vi "ME35.vi"() -> ()   [LabVIEW 2020]
panel:
  in  "Tab Control":T1(tab)
  in  "ports":bool
  in  "Prefs":bool
  in  "FileUpload":bool
  in  "VI Examples":u16(ring) items=["01 Controls and Indicators.vi", "02 Tools, Colors, and Clicks.vi", "03 Charts.vi", "04 Loops.vi", "05 Graphs.vi", "06 Shift Registers.vi", "07 Arrays.vi", "08 Strings.vi", "09 Clusters.vi", "10 Rings, Strings, and Tables.vi", "11 Execution Order.vi", "12 Events.vi", "13 Case Structures.vi", "14 Saving and Reading Files.vi", "15 Messing with Time.vi", "16 JSON Packets.vi", "21 Talking Serial.vi", "22 RESTful API.vi", "23 Python Node.vi", "24 OS Commands.vi", "51 Simple Queues.vi", "52 Properties.vi", "53 Invoke.vi", "54 Occurences and more.vi", "55 Channels.vi", "56 Panels in panels.vi", "57 Scripting.vi", "71 MP_Reading a voltage.vi", "72 MP_Setting a servo.vi", "81 Arduino_Reading a voltage.vi", "82 Arduino_Setting a servo.vi", "91 WIO_Reading a voltage.vi", "92 WIO_Setting a Servo.vi"]
  in  "VIs":bool
  in  "rPi":bool
  in  "IP Address":string
  in  "WIO":bool
  in  "WIO Port":string(combo)
  in  "Connect":bool
  in  "Port":string(combo)
  out "Python version":string="3.9"
  out "OUTPUT CONSOLE":string
  in  "Home 2":bool
  in  "Prefs":T2={"Python version"="3.9", "arduino15"=path "", "arduino Lib"=path ""}
  in  "Home":bool
  # "ME35\nversion 0.1b02"
  # "This program uses python codes under the hood to talk over the serial port, over SSH, and to cameras.  You should using version 3.6 or later and should have pyserial installed."
  # "This is the path to your Arduino app.  Click on the folder icon and select the app."
  # "This is the path to your Arduinolibarry folder (typically in your documents folder)"
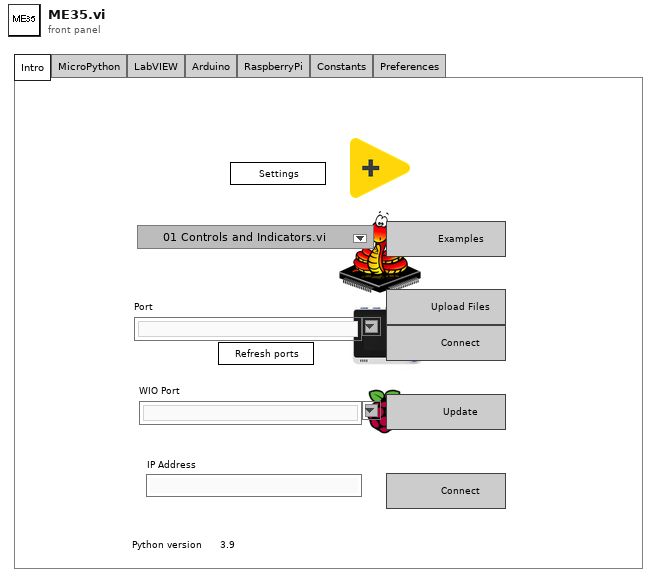
[diagram p1: front panel]
types:
  T1 = enum32{"Intro", "MicroPython", "LabVIEW", "Arduino", "RaspberryPi", "Constants", "Preferences"}
  T2 = cluster{"Python version":string, "arduino15":path, "arduino Lib":path}
  T3 = enum32{"Invalid", "Standard", "Closed", "Hidden", "Minimized", "Maximized"}
  T4 = typedef "Preferences.ctl" = cluster{"python":string, "arduino15":path, "arduino Lib":path}
  T5 = typedef "PythonCtrl.ctl" = cluster{"session":refnum<k35>, "PyPath":path}
  T6 = typedef "Arduino.ctl" = cluster{"Java":path, "Packages":path, "folder":path, "serial":string, "Console":string}
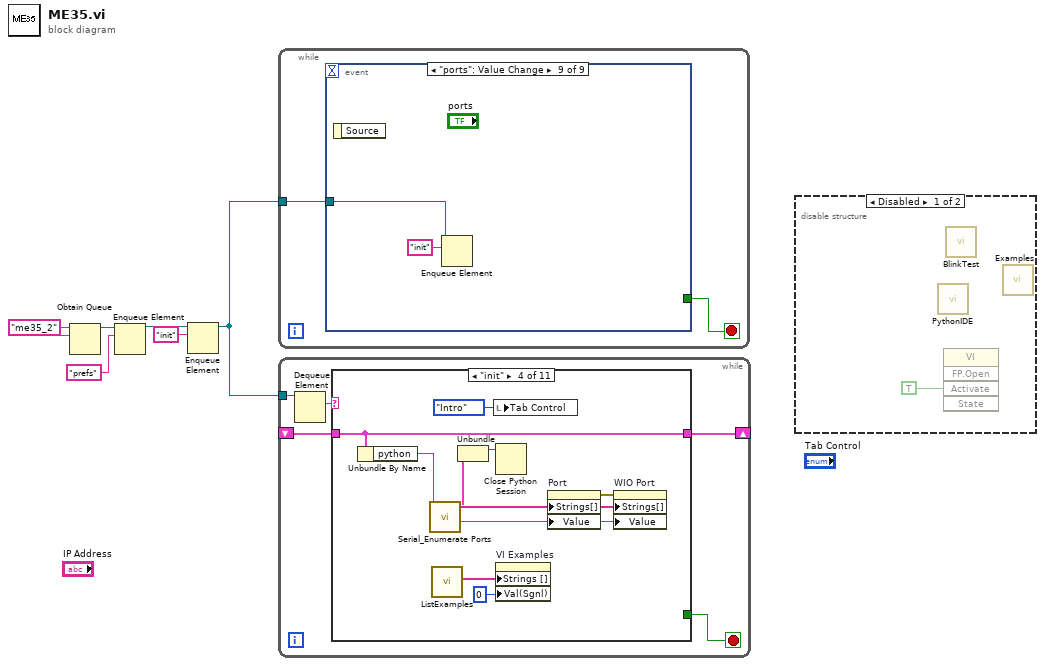
[diagram p0: block diagram]
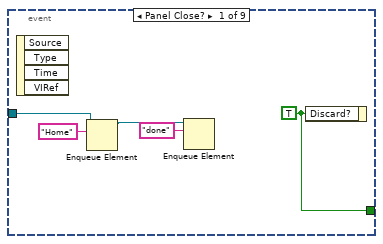
[diagram p3: hidden frame]
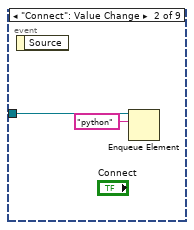
[diagram p4: hidden frame]
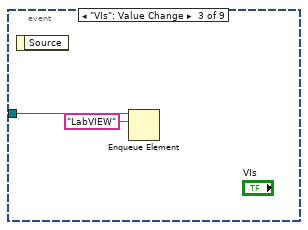
[diagram p5: hidden frame]
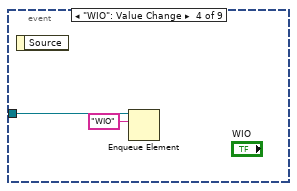
[diagram p6: hidden frame]
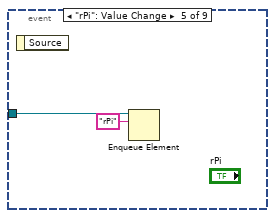
[diagram p7: hidden frame]
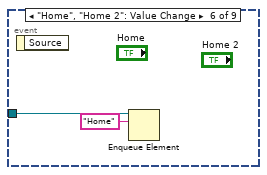
[diagram p8: hidden frame]
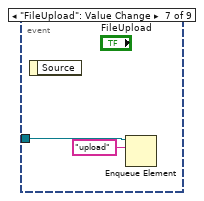
[diagram p9: hidden frame]
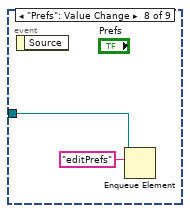
[diagram p10: hidden frame]
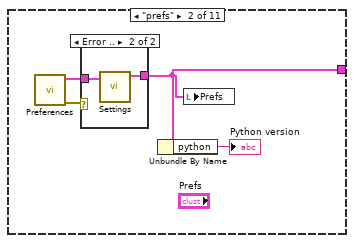
[diagram p12: hidden frame]
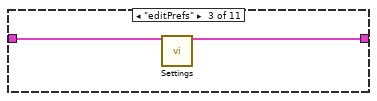
[diagram p14: hidden frame]
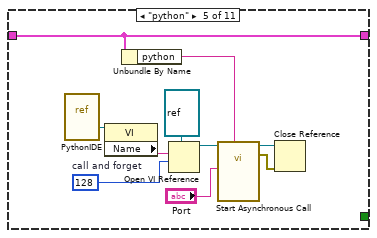
[diagram p15: hidden frame]
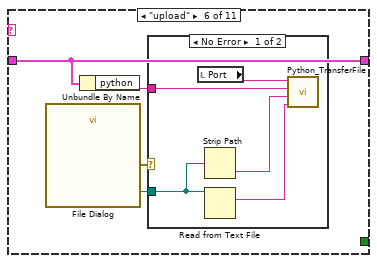
[diagram p16: hidden frame]
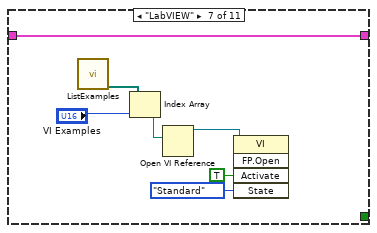
[diagram p18: hidden frame]
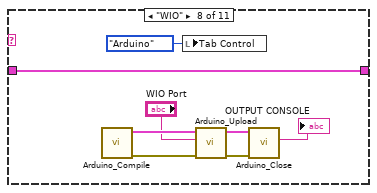
[diagram p19: hidden frame]
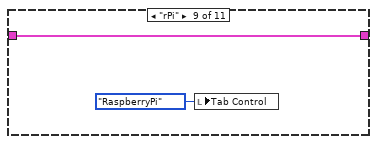
[diagram p20: hidden frame]
diagram:
  w6 = "me35_2" ("name (unnamed)")
  n1 = Obtain Queue(name (unnamed)=w6, element data type=w6) -> (queue out=w2:refnum<queue>)  [unwired: 3 in, 2 out]
  n2 = Enqueue Element(queue=w2, element="prefs") -> (queue out=w1:refnum<queue>)  [unwired: 2 in, 2 out]
  n3 = Enqueue Element(queue=w1, element="init") -> (queue out=w5:refnum<queue>)  [unwired: 2 in, 2 out]
  n4 = while {
    tunnel: w5 -> [w8]
    stop <- w7 stop-if-true
    n5 = event shown="[8] \"ports\": Value Change" {
      selector: _ -> [_ _ _ _ _ _ _ _ _]
      dyn-events: _ -> [_ _ _ _ _ _ _ _ _]
      timeout: _ -> [_ _ _ _ _ _ _ _ _]
      tunnel: w8 -> [w10 w15 w17 w19 w21 w23 w24 w26 w28]
      tunnel: [w13 _ _ _ _ _ _ _ _] -> w7
      event Panel Close? {
        w13 = TRUE ("Discard?")
        n6 = event-data() -> ()  [unwired: 1 in, 4 out]
        n7 = Enqueue Element(queue=w10, element="Home") -> (queue out=w9:refnum<queue>)  [unwired: 2 in, 2 out]
        n8 = Enqueue Element(queue=w9, element="done") -> ()  [unwired: 2 in, 3 out]
        n9 = event-data("Discard?"=w13) -> ()  [unwired: 1 in, 1 out]
      }
      event "Connect": Value Change {
        n10 = event-data() -> ()  [unwired: 1 in, 1 out]
        n11 = Enqueue Element(queue=w15, element="python") -> ()  [unwired: 2 in, 3 out]
      }
      event "VIs": Value Change {
        n12 = event-data() -> ()  [unwired: 1 in, 1 out]
        n13 = Enqueue Element(queue=w17, element="LabVIEW") -> ()  [unwired: 2 in, 3 out]
      }
      event "WIO": Value Change {
        n14 = event-data() -> ()  [unwired: 1 in, 1 out]
        n15 = Enqueue Element(queue=w19, element="WIO") -> ()  [unwired: 2 in, 3 out]
      }
      event "rPi": Value Change {
        n16 = event-data() -> ()  [unwired: 1 in, 1 out]
        n17 = Enqueue Element(queue=w21, element="rPi") -> ()  [unwired: 2 in, 3 out]
      }
      event "Home", "Home 2": Value Change {
        n18 = event-data() -> ()  [unwired: 1 in, 1 out]
        n19 = Enqueue Element(queue=w23, element="Home") -> ()  [unwired: 2 in, 3 out]
      }
      event "FileUpload": Value Change {
        n20 = event-data() -> ()  [unwired: 1 in, 1 out]
        n21 = Enqueue Element(queue=w24, element="upload") -> ()  [unwired: 2 in, 3 out]
      }
      event "Prefs": Value Change {
        n22 = event-data() -> ()  [unwired: 1 in, 1 out]
        n23 = Enqueue Element(queue=w26, element="editPrefs") -> ()  [unwired: 2 in, 3 out]
      }
      event "ports": Value Change {
        n24 = event-data() -> ()  [unwired: 1 in, 1 out]
        n25 = Enqueue Element(queue=w28, element="init") -> ()  [unwired: 2 in, 3 out]
      }
    }
  }
  n26 = while {
    tunnel: w5 -> [w34]
    shift-right: [w31] -> _
    shift-left: _ -> [w30]
    stop <- w32 stop-if-true
    n27 = Dequeue Element(queue=w34) -> (element=w33:string)  [unwired: 2 in, 3 out]
    n28 = case shown="\"init\"" w33 {
      tunnel: [_ _ _ _ _ _ _ _ _ _ TRUE ("Discard?")] -> w32
      tunnel: [w35 w36 w43 w45 w56 w68 w74 w81 w89 w91 w93] -> w31
      tunnel: w30 -> [w35 _ w44 w45 w56 w68 w74 w81 w89 w91 w93]
      frame Default {
      }
      frame "prefs" {
        n29 = call "Preferences.vi"() -> ("error out"=w38:errorcluster, "Preferences out"=w37:T4)  [unwired: 10 in]
        n30 = case shown="Error .." w38 {
          tunnel: w37 -> [w40 w42]
          tunnel: [w40 w41] -> w36
          frame No Error {
          }
          frame Error {
            n31 = call "Settings.vi"("Prefs"=w42) -> ("Preferences"=w41:T4)  [unwired: 10 in]
          }
        }
        n32 = Unbundle By Name(w36) -> ("python"=→"Python version":string)
        n33 = local write "Prefs"(w36) -> ()
      }
      frame "editPrefs" {
        n34 = call "Settings.vi"("Prefs"=w44) -> ("Preferences"=w43:T4)  [unwired: 10 in]
      }
      frame "init" {
        n35 = Unbundle By Name(w45) -> ("python"=w47:string)
        n36 = call "Serial_Enumerate Ports.vi"("Python version"=w47) -> ("guess"=w54:string, "Python"=w51:T5, "possibilities"=w53:string[])  [unwired: 7 in, 1 out]
        n37 = call "ListExamples.vi"() -> ("vis"=w50:string[])  [unwired: 7 in, 4 out]
        n38 = Unbundle(w51) -> ("session"=w48:refnum<k35>)  [unwired: 1 out]
        n39 = local write "Tab Control"(T1."Intro" ("Tab Control")) -> ()
        n40 = Close Python Session(session in=w48) -> ()  [unwired: 1 in, 1 out]
        n41 = property on="VI Examples" class="Ring (strict)"("Strings []"=w50, "Val(Sgnl)"=u16 0 ("Value (Signaling)")) -> ()  [unwired: 2 in, 2 out]
        n42 = property on="Port" class="CmbBox"("Strings[]"=w53, "Value"=w54) -> (error out=w52:errorcluster)  [unwired: 2 in, 1 out]
        n43 = property on="WIO Port" class="CmbBox"(error in=w52, "Strings[]"=w53, "Value"=w54) -> ()  [unwired: 1 in, 2 out]
      }
      frame "python" {
        w63 = 128  # call and forget
        n44 = vi-ref "PythonIDE.vi"() -> (w59:refnum<vi>)
        n45 = property class="VI"(reference=w59) -> ("Name"=w60:string)  [unwired: 1 in, 2 out]
        n46 = Unbundle By Name(w56) -> ("python"=w55:string)
        n47 = Open VI Reference(type specifier VI Refnum (for type only)=refnum<vi> refnum, vi path=w60, options=w63) -> (vi reference=w64:refnum<vi>)  [unwired: 3 in, 1 out]
        n48 = call-by-ref "Start Asynchronous Call"(reference=w64, "Python version"=w55, "Port"="Port") -> (reference out=w57:refnum<vi>, error out=w58:errorcluster)  [unwired: 11 in]
        n49 = Close Reference(reference=w57, error in (no error)=w58) -> ()  [unwired: 1 out]
      }
      frame "upload" {
        n50 = call "File Dialog"() -> ("selected path"=w66:path, "error out"=w65:errorcluster)  [unwired: 12 in, 2 out]
        n51 = Unbundle By Name(w68) -> ("python"=w67:string)
        n52 = case shown="No Error" w65 {
          tunnel: w66 -> [w70 _]
          tunnel: w67 -> [w69 _]
          frame No Error {
            n53 = local read "Port"() -> (w73:string)
            n54 = Strip Path(path=w70) -> (name=w71:string)  [unwired: 1 out]
            n55 = Read from Text File(file (use dialog)=w70) -> (text=w72:string)  [unwired: 3 in, 3 out]
            n56 = call "Python_TransferFile.vi"("File text"=w72, "File name"=w71, "Python version"=w69, "Port"=w73) -> ()  [unwired: 7 in, 1 out]
          }
          frame Error {
          }
        }
      }
      frame "LabVIEW" {
        n57 = call "ListExamples.vi"() -> ("VI Paths"=w78:path[])  [unwired: 7 in, 4 out]
        n58 = Index Array(array=w78, index="VI Examples") -> (element=w80:path)
        n59 = Open VI Reference(vi path=w80) -> (vi reference=w77:refnum<vi>)  [unwired: 5 in, 1 out]
        n60 = invoke class="VI" method="FP.Open"(reference=w77, "Activate"=TRUE ("Activate?"), "State"=T3."Standard") -> ()  [unwired: 2 in, 5 out]
      }
      frame "WIO" {
        n61 = call "Arduino_Compile.vi"() -> ("error out"=w87:errorcluster, "Arduino Out"=w85:T6)  [unwired: 10 in]
        n62 = local write "Tab Control"(T1."Arduino" ("Tab Control")) -> ()
        n63 = call "Arduino_Upload.vi"("error in (no error)"=w87, "serial"="WIO Port", "Arduino In"=w85) -> ("error out"=w86:errorcluster, "Arduino Out"=w84:T6)  [unwired: 7 in]
        n64 = call "Arduino_Close.vi"("error in (no error)"=w86, "Arduino In"=w84) -> ("Console"=→"OUTPUT CONSOLE":string)  [unwired: 8 in, 1 out]
      }
      frame "rPi" {
        n65 = local write "Tab Control"(T1."RaspberryPi" ("Tab Control")) -> ()
      }
      frame "Home" {
        n66 = local write "Tab Control"(T1."Intro" ("Tab Control")) -> ()
      }
      frame "done" {
      }
    }
  }
  n67 = disable-structure shown="Disabled" {
    frame Disabled {
      n68 = call "PythonIDE.vi"() -> ()  [unwired: 12 in]
      n69 = invoke class="VI" method="FP.Open"("Activate"=TRUE ("Activate?")) -> ()  [unwired: 4 in, 5 out]
      n70 = call "BlinkTest.vi"() -> ()  [unwired: 12 in]
      n71 = call "Examples.vi"() -> ()  [unwired: 12 in]
    }
    frame Enabled {
    }
  }
